vi "simulaFrec.vi"(8 "error in (no error)":errorcluster, 10 "frec in":dbl=0.75 format="%#_13g") -> (0 "error out":errorcluster, 2 "frec out":dbl, 3 "Keithley2002 out":refnum<class "Keithley2002.lvclass">)   [LabVIEW 2019, in "CNT90.lvclass"]
uses:
  CNT90.lvclass
  Keithley2002/Keithley2002.lvclass
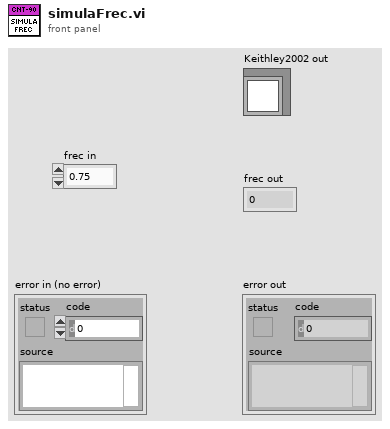
[diagram p1: front panel]
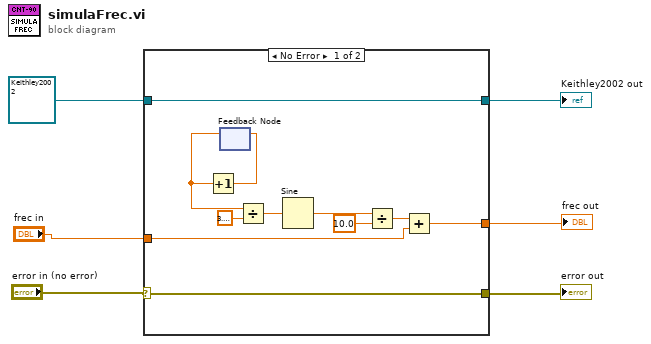
[diagram p0: block diagram]
diagram:
  n1 = case shown="No Error" "error in (no error)" {
    selector: "error in (no error)" -> [w10 w18]
    tunnel: [w10 w18] -> w5
    tunnel: [w9 w19] -> w4
    tunnel: refnum<class "Keithley2002.lvclass"> refnum ("Keithley2002 in") -> [w9 w19]
    tunnel: "frec in" -> [w8 _]
    tunnel: [w7 _] -> w1
    frame No Error {
      n2 = feedback #1() -> (w13:dbl)  [unwired: 1 in]
      n3 = Increment(x=w13) -> (x+1=w17:dbl)
      n4 = feedback-in #1(w17) -> ()
      n5 = Divide(x=w13, y=3.141592653589793) -> (x/y=w16:dbl)
      n6 = Sine(x=w16) -> (sin(x)=w14:dbl)
      n7 = Divide(x=w14, y=10.0) -> (x/y=w12:dbl)
      n8 = Add(x=w12, y=w8) -> (x+y=w7:dbl)
    }
    frame Error {
    }
  }
  "error out" <- w5
  "Keithley2002 out" <- w4
  "frec out" <- w1
